vi "FTW-VIServer-GetClassDefaultData.vi"(0 "Fully-Qualified Class Name":string, 11 "error in":errorcluster) -> (4 "Class Data":string, 6 "Class Version":string, 15 "error out":errorcluster)   [LabVIEW 2013]
uses:
  Error/FTW-ERR-ThrowError.vi
panel:
  # "Inputs"
  # "Outputs"
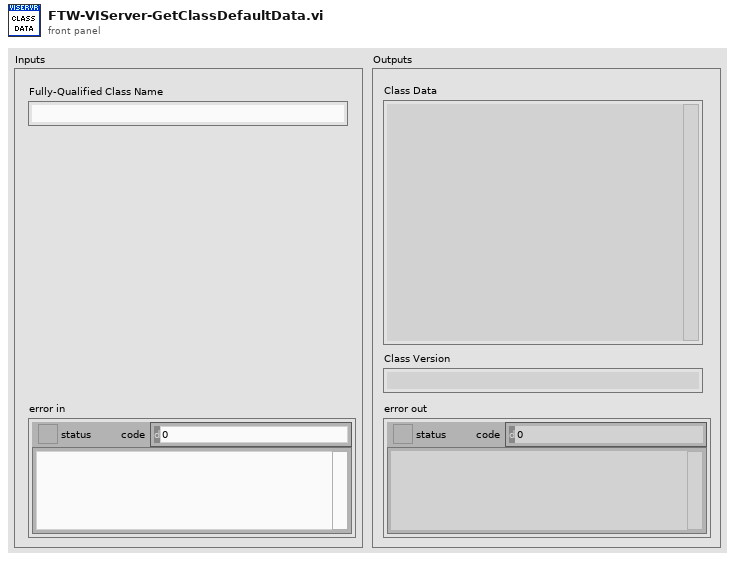
[diagram p1: front panel]
types:
  T1 = cluster{"Major":u16, "Minor":u16, "Fix":u16, "Build":u16}
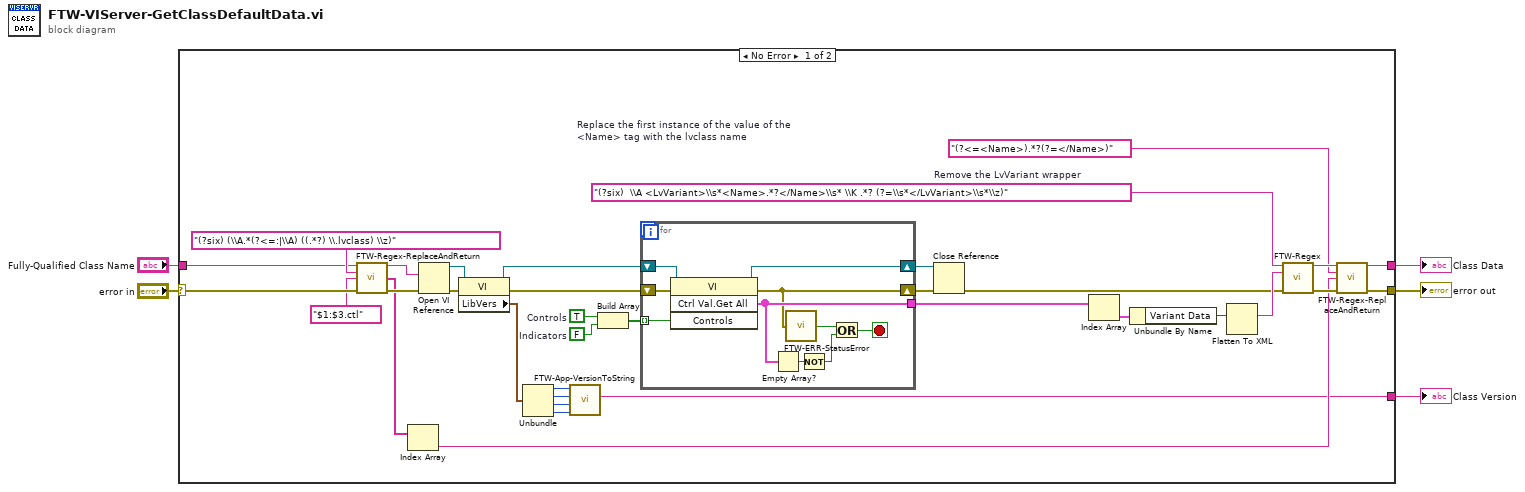
[diagram p0: block diagram]
diagram:
  n1 = case shown="No Error" "error in" {
    selector: "error in" -> [w32 w50]
    tunnel: [w17 w50] -> w4
    tunnel: "Fully-Qualified Class Name" -> [w21 _]
    tunnel: [w18 _] -> w2
    tunnel: [w6 _] -> w1
    frame No Error {
      w25 = "(?<=<Name>).*?(?=</Name>)"  # Replace the first instance of the value of the <Name> tag with the lvclass name
      w30 = "(?six)  \\A <LvVariant>\\s*<Name>.*?</Name>\\s* \\K .*? (?=\\s*</LvVariant>\\s*\\z)"  # Remove the LvVariant wrapper
      w37 = FALSE  # Indicators
      w38 = TRUE  # Controls
      n2 = call "FTW-Regex-ReplaceAndReturn.vi"("String"=w21, "Search for (Regular Expression)"="(?six) (\\A.*(?<=:|\\A) ((.*?) \\.lvclass) \\z)", "Replace with"="$1:$3.ctl", "error in"=w32) -> ("String out"=w33:string, "Submatches"=w20:string[], "error out"=w22:errorcluster)  [unwired: 7 in, 2 out]
      n3 = Index Array(array=w20) -> (element=w19:string)  [unwired: 1 in]
      n4 = Open VI Reference(vi path=w33, error in (no error)=w22) -> (vi reference=w15:refnum<vi>, error out=w13:errorcluster)  [unwired: 4 in]
      n5 = property class="VI"(reference=w15, error in=w13) -> (reference out=w14:refnum<vi>, error out=w12:errorcluster, "LibVers"=w11:T1)
      n6 = Unbundle(w11) -> ("Major"=w10:u16, "Minor"=w9:u16, "Fix"=w8:u16, "Build"=w7:u16)
      n7 = call "FTW-App-VersionToString.vi"("Build"=w7, "Fix"=w8, "Minor"=w9, "Major"=w10) -> ("Version String"=w6:string)  [unwired: 6 in, 1 out]
      n8 = Build Array(w38, w37) -> (w39:bool[])
      n9 = for {
        shift-right: [w41] -> w29
        shift-left: w12 -> [w48]
        tunnel: w39 -> [w47] mode=indexing
        tunnel: [w43] -> w36
        shift-right: [w40] -> w16
        shift-left: w14 -> [w49]
        stop <- w42 stop-if-true
        n10 = invoke class="VI" method="Ctrl Val.Get All"(reference=w49, error in=w48, "Controls"=w47) -> (reference out=w40:refnum<vi>, error out=w41:errorcluster, "Get All Control Values Variant"=w43:cluster{"Name":string, "Variant Data":variant}[])  [unwired: 1 in, 1 out]
        n11 = Empty Array?(array=w43) -> (empty?=w45:bool)
        n12 = call "FTW-ERR-StatusError.vi"("error to check"=w41) -> ("Error?"=w46:bool)
        n13 = Not(x=w45) -> (.not. x?=w44:bool)
        n14 = Or(x=w46, y=w44) -> (x .or. y?=w42:bool)
      }
      n15 = Close Reference(reference=w16, error in (no error)=w29) -> (error out=w28:errorcluster)
      n16 = Index Array(array=w36) -> (element=w35:cluster{"Name":string, "Variant Data":variant})  [unwired: 1 in]
      n17 = Unbundle By Name(w35) -> ("Variant Data"=w34:variant)
      n18 = Flatten To XML(anything=w34) -> (xml string=w31:string)
      n19 = call "FTW-Regex.vi"("Regular Expression"=w30, "Input String"=w31, "error in"=w28) -> ("Match"=w27:string, "error out"=w26:errorcluster)  [unwired: 8 in, 3 out]
      n20 = call "FTW-Regex-ReplaceAndReturn.vi"("String"=w27, "Search for (Regular Expression)"=w25, "Replace with"=w19, "error in"=w26) -> ("String out"=w18:string, "error out"=w17:errorcluster)  [unwired: 7 in, 3 out]
    }
    frame Error {
    }
  }
  "error out" <- w4
  "Class Data" <- w2
  "Class Version" <- w1
